vi "Create.vi"(8 "error in (no error)":errorcluster, 10 "Serial":refnum<class "Serial.lvclass">) -> (0 "error out":errorcluster, 3 "Driver":refnum<class "Driver.lvclass">)   [LabVIEW 2020, in "Driver.lvclass"]
uses:
  Driver.lvclass
  Serial/Serial.lvclass/Serial.lvclass
  Driver.lvclass/Driver.ctl
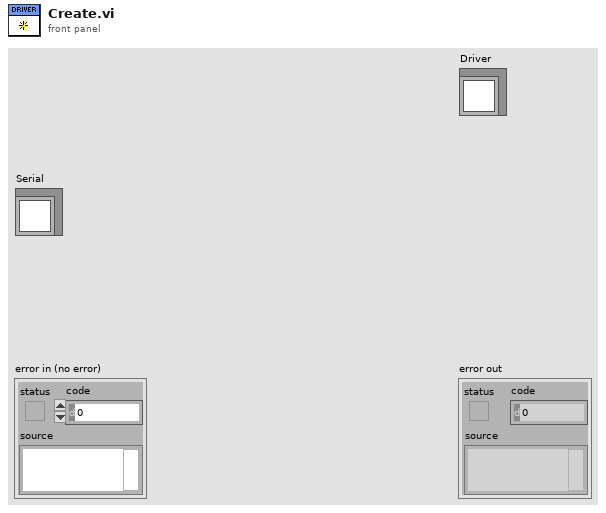
[diagram p1: front panel]
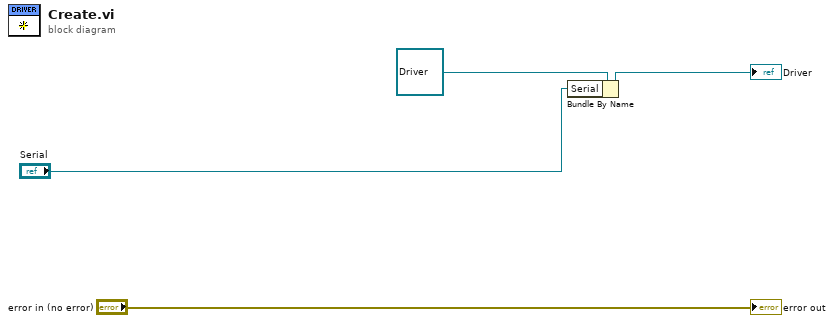
[diagram p0: block diagram]
diagram:
  n1 = Bundle By Name(cluster=refnum<class "Driver.lvclass"> refnum ("Driver"), "Serial"="Serial") -> (→"Driver":refnum<class "Driver.lvclass">)
  "error out" <- "error in (no error)"
